vi "Initial Vectors Calc.vi"(0 "Catapult Move\nAngle":dbl, 5 "Time of Rotation":dbl) -> (1 "2D Plot Class Obj Array out":refnum<class "2D Plot Datatype.lvclass">[](array[class]), 4 "X Initial distance from ultrasonic":dbl, 6 "Y Initial distance from ultrasonic":dbl, 8 "Angular Velocity":dbl, 10 "X Delta (m)":dbl, 12 "Angle of Throw Relative to Forward Horizantal = 0":dbl, 13 "Angle of Throw":dbl, 14 "Angle of Catapult":dbl, 15 "Y Delta (m)":dbl)   [LabVIEW 2013]
uses:
  <vilib>/Math Plots/2D Math Plots/2D Compass/2D Compass XCtrl/2D Compass.xctl
  <vilib>/Math Plots/2D Math Plots/2D Plot/2D Plot Datatype/2D Plot Datatype.lvclass
  <vilib>/Math Plots/2D Math Plots/2D Compass/2D Compass Datatype/Public/Plot Helper (Vector).vi
  <vilib>/Math Plots/2D Math Plots/2D Compass/2D Compass Datatype/2D Compass Datatype.lvclass
panel:
  out "Initial Throw Angle":refnum<class "2D Plot Datatype.lvclass">[](xcontrol) caption="2D Compass"
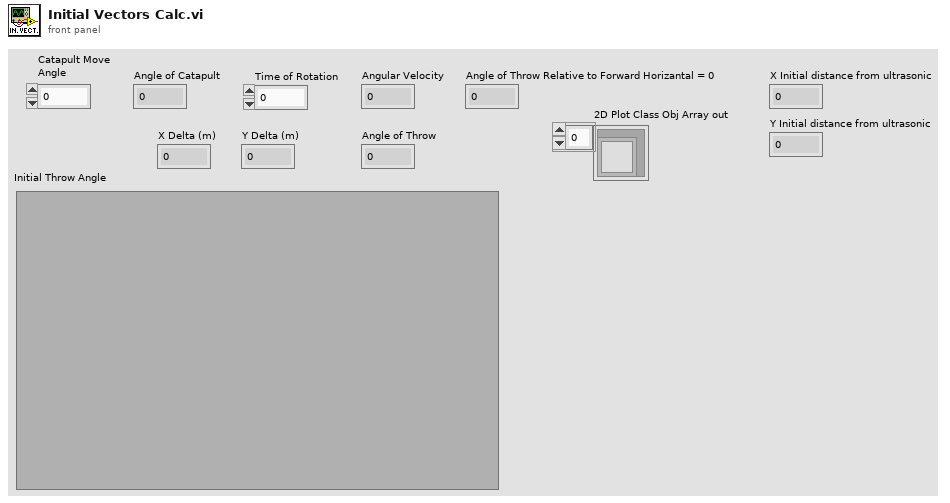
[diagram p1: front panel]
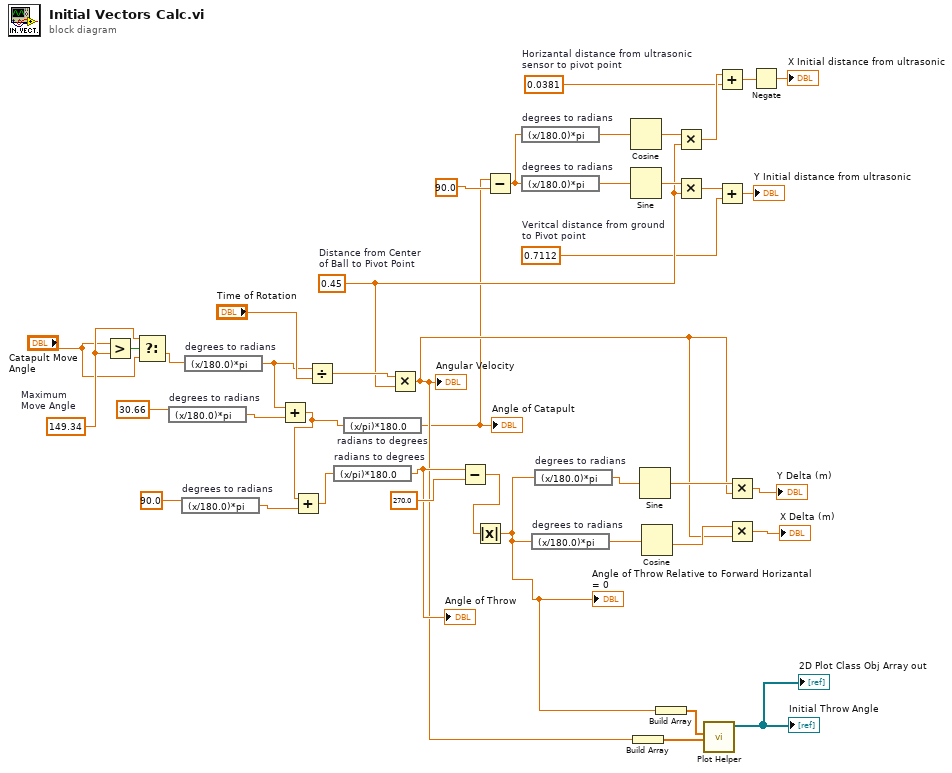
[diagram p0: block diagram]
diagram:
  w9 = 0.45  # Distance from Center of Ball to Pivot Point
  w5 = 0.0381  # Horizantal distance from ultrasonic sensor to pivot point
  w6 = 0.7112  # Veritcal distance from ground to Pivot point
  w21 = 149.34  # Maximum Move Angle
  n1 = Greater?(x="Catapult Move\nAngle", y=w21) -> (0:w22:bool)
  n2 = Select(t=w21, s=w22, f="Catapult Move\nAngle") -> (s? t:f=w20:dbl)
  n3 = expression code="(x/180.0)*pi" "degrees to radians"(30.66 ("y")) -> (w39:dbl)
  n4 = expression code="(x/180.0)*pi" "degrees to radians"(90.0 ("y")) -> (w31:dbl)
  n5 = expression code="(x/180.0)*pi" "degrees to radians"(w20) -> (w38:dbl)
  n6 = Add(x=w38, y=w39) -> (x+y=w28:dbl)
  n7 = Add(x=w28, y=w31) -> (x+y=w29:dbl)
  n8 = Divide(x=w38, y="Time of Rotation") -> (x/y=w41:dbl)
  n9 = expression code="(x/pi)*180.0" "radians to degrees"(w29) -> (w27:dbl)
  "Angle of Throw" <- w27
  n10 = expression code="(x/pi)*180.0" "radians to degrees"(w28) -> (w3:dbl)
  "Angle of Catapult" <- w3
  n11 = Multiply(x=w41, y=w9) -> (x*y=w24:dbl)
  "Angular Velocity" <- w24
  n12 = Subtract(x=w27, y=270.0) -> (x-y=w32:dbl)
  n13 = Absolute Value(x=w32) -> (abs(x)=w18:dbl)
  "Angle of Throw Relative to Forward Horizantal = 0" <- w18
  n14 = Subtract(x=w3, y=90.0) -> (x-y=w12:dbl)
  n15 = expression code="(x/180.0)*pi" "degrees to radians"(w12) -> (w14:dbl)
  n16 = expression code="(x/180.0)*pi" "degrees to radians"(w12) -> (w13:dbl)
  n17 = expression code="(x/180.0)*pi" "degrees to radians"(w18) -> (w25:dbl)
  n18 = expression code="(x/180.0)*pi" "degrees to radians"(w18) -> (w26:dbl)
  n19 = Cosine(x=w14) -> (cos(x)=w10:dbl)
  n20 = Sine(x=w13) -> (sin(x)=w11:dbl)
  n21 = Build Array(w24) -> (w23:dbl[])
  n22 = Sine(x=w26) -> (sin(x)=w34:dbl)
  n23 = Cosine(x=w25) -> (cos(x)=w36:dbl)
  n24 = Build Array(w18) -> (w17:dbl[])
  n25 = Multiply(x=w10, y=w9) -> (x*y=w7:dbl)
  n26 = Multiply(x=w11, y=w9) -> (x*y=w8:dbl)
  n27 = call-poly <vilib>:"Plot Helper.vi"("radius vector"=w23, "theta vector"=w17) -> ("2D Plot Class Obj Array out"=→"Initial Throw Angle" →"2D Plot Class Obj Array out":refnum<class "2D Plot Datatype.lvclass">[])  [unwired: 2 in, 7 out]
  n28 = Add(x=w7, y=w5) -> (x+y=w2:dbl)
  n29 = Add(x=w8, y=w6) -> (x+y=→"Y Initial distance from ultrasonic":dbl)
  n30 = Multiply(x=w34, y=w24) -> (x*y=→"Y Delta (m)":dbl)
  n31 = Multiply(x=w36, y=w24) -> (x*y=→"X Delta (m)":dbl)
  n32 = Negate(x=w2) -> (-x=→"X Initial distance from ultrasonic":dbl)
